vi "DHE_InitGeometry.vi"(0 "refnum":i32=2048, 1 "override format":string, 11 "error in (no error)":errorcluster, 12 "Database RefNum out":T1, 13 "forece init":bool) -> (4 "fd out":i32, 6 "return value":i32, 8 "X total size":u16, 10 "Y total size":u16, 14 "DET_READ_TIME":sgl=3.5 format="%.6f", 15 "error out":errorcluster)   [LabVIEW 2016]
uses:
  DBSHAND/private/vis/DatabaseHand_RefNum.ctl
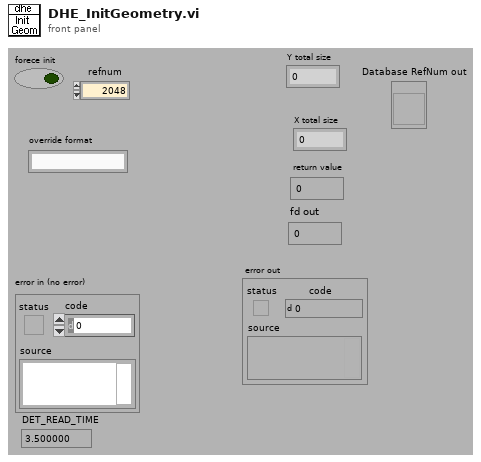
[diagram p1: front panel]
types:
  T1 = typedef "DatabaseHand_RefNum.ctl" = refnum<vi>
  T2 = cluster{"Video Processor Type":string, "support gain":bool, "Timing Board":string, "support reset":bool, "Utility Board":string, "Shutter":string, "Temperature":string, "support temp control":bool, "Detector Type":string, "Support MPP":string, "Support Binning":string, "Readout Mode":string, "support shutter control":bool}
  T3 = typedef "GEOM_CorrectedFPA.ctl" = cluster{"readmode":string, "amplifiers":cluster{"number":i32, "xstart":i32, "ystart":i32}[], "totxsize":i32, "totysize":i32, "maxxdim":i32, "maxydim":i32, "numxamps":i32, "numyamps":i32, "totxdata":i32, "totydata":i32, "xdataamp":i32, "ydataamp":i32, "totpixels":i32}
  T4 = typedef "GEOM_Amplifier.ctl" = cluster{"number":i32, "type":T5, "rotated":i16, "fliped":u16, "FPAcoord":cluster{"xstart":i32, "ystart":i32}, "Physical_size":cluster{"columns":i32, "rows":i32}, "predata":cluster{"columns":i32, "rows":i32}, "postdata":cluster{"columns":i32, "rows":i32}, "Req ROIs":T6, "Corr ROI":T6, "Detnumber":i32, "ampID":string, "discard":i32}
  T5 = typedef "GEOM_AmpType.ctl" = u16
  T6 = typedef "GEOM_ROI.ctl" = T7[]
  T7 = typedef "GEOM_Coords.ctl" = cluster{"xstart":u32, "ystart":u32, "xsize":u32, "ysize":u32}
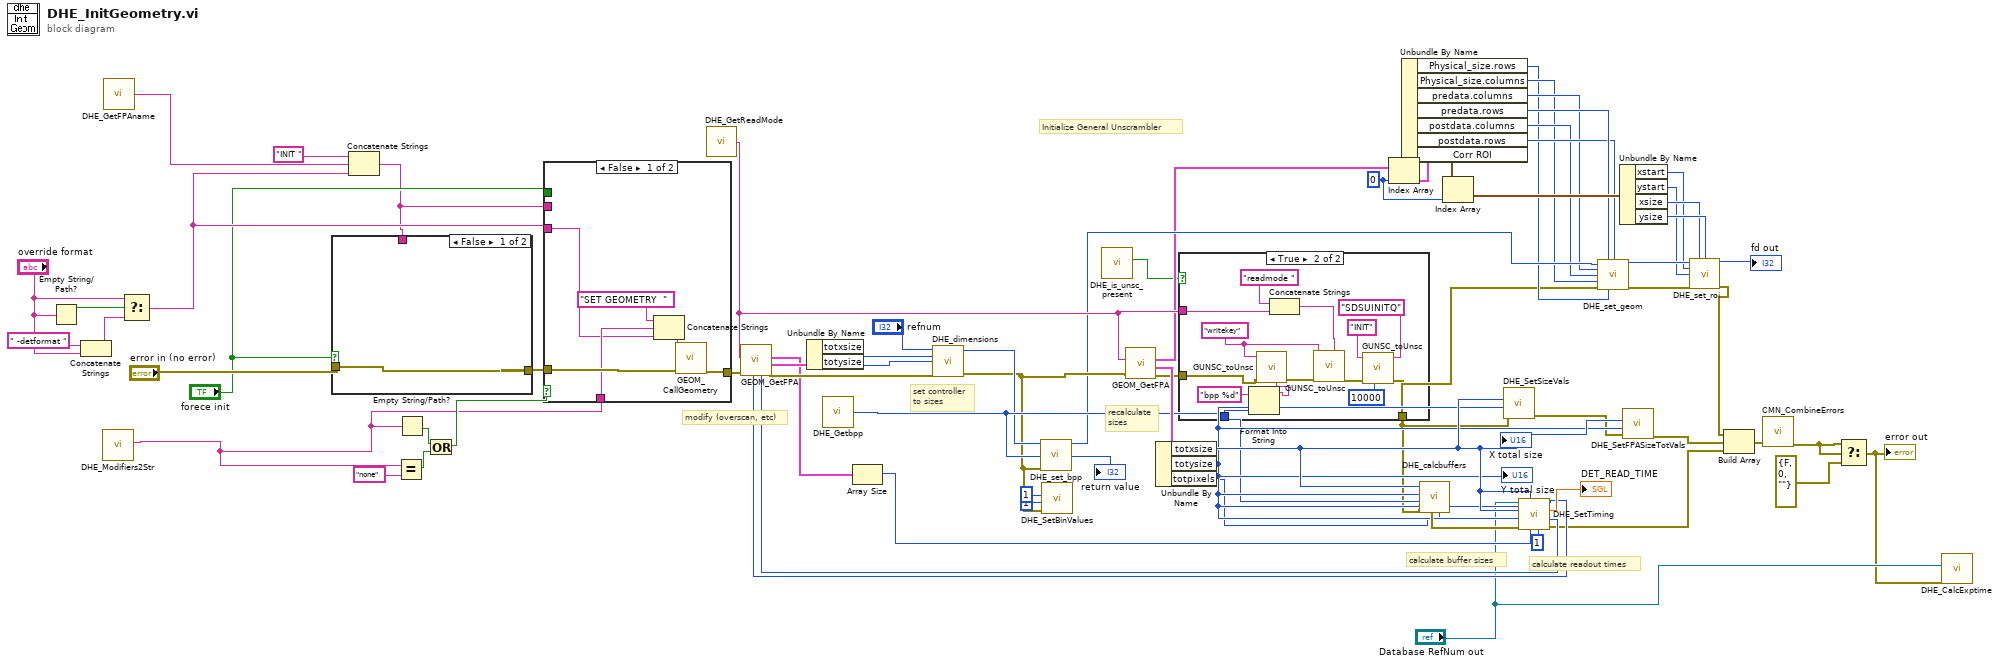
[diagram p0: block diagram]
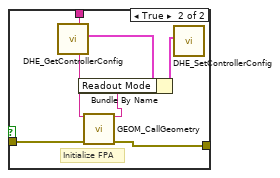
[diagram p2: hidden frame]
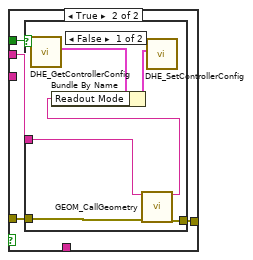
[diagram p4: hidden frame]
diagram:
  w35 = 0 ("index")
  # "calculate readout times"
  # "calculate buffer sizes"
  # "Initialize General Unscrambler"
  # "recalculate\nsizes"
  # "set controller\nto sizes"
  # "modify (overscan, etc)"
  n1 = Empty String/Path?(string/path="override format") -> (empty?=w46:bool)
  n2 = Concatenate Strings(" -detformat " ("string"), "override format") -> (w43:string)
  n3 = call "DHE_Modifiers2Str.vi"() -> ("modifiers"=w4:string)  [unwired: 11 out]
  n4 = call "DHE_GetFPAname.vi"() -> ("DHE_FPAname"=w42:string)  [unwired: 9 out]
  n5 = Select(t="override format", s=w46, f=w43) -> (s? t:f=w36:string)
  n6 = Concatenate Strings("INIT " ("string"), w42, w36) -> (w5:string)
  n7 = case shown="False" "forece init" {
    tunnel: "error in (no error)" -> [w72 w78]
    tunnel: [w72 w77] -> w7
    tunnel: w5 -> [_ w76]
    frame False {
    }
    frame True {
      # "Initialize FPA"
      n8 = call "DHE_GetControllerConfig.vi"() -> ("ControllerConfigCluster"=w74:T2)  [unwired: 11 out]
      n9 = call "GEOM_CallGeometry.vi"("Command"=w76, "error in (no error)"=w78) -> ("ImmedReplyString"=w73:string, "error out"=w77:errorcluster)  [unwired: 12 out]
      n10 = Bundle By Name(cluster=w74, "Readout Mode"=w73) -> (w75:T2)
      n11 = call "DHE_SetControllerConfig.vi"("ControllerConfigCluster"=w75) -> ()  [unwired: 11 out]
    }
  }
  n12 = Equal?(x=w4, y="none") -> (x = y?=w59:bool)
  n13 = Empty String/Path?(string/path=w4) -> (empty?=w60:bool)
  n14 = Or(x=w60, y=w59) -> (x .or. y?=w58:bool)
  n15 = case shown="False" w58 {
    tunnel: w7 -> [w84 w88]
    tunnel: [w81 w87] -> w70
    tunnel: w4 -> [w80 _]
    tunnel: w36 -> [w79 _]
    tunnel: w5 -> [_ w86]
    tunnel: "forece init" -> [_ w85]
    frame False {
      n16 = Concatenate Strings("SET GEOMETRY  " ("Command"), w80, w79) -> (w82:string)
      n17 = call "GEOM_CallGeometry.vi"("Command"=w82, "error in (no error)"=w84) -> ("error out"=w81:errorcluster)  [unwired: 13 out]
    }
    frame True {
      n18 = case shown="False" w85 {
        tunnel: w88 -> [w94 w95]
        tunnel: [w93 w95] -> w87
        tunnel: w86 -> [w92 _]
        frame False {
          n19 = call "DHE_GetControllerConfig.vi"() -> ("ControllerConfigCluster"=w91:T2)  [unwired: 11 out]
          n20 = call "GEOM_CallGeometry.vi"("Command"=w92, "error in (no error)"=w94) -> ("ImmedReplyString"=w89:string, "error out"=w93:errorcluster)  [unwired: 12 out]
          n21 = Bundle By Name(cluster=w91, "Readout Mode"=w89) -> (w90:T2)
          n22 = call "DHE_SetControllerConfig.vi"("ControllerConfigCluster"=w90) -> ()  [unwired: 11 out]
        }
        frame True {
        }
      }
    }
  }
  n23 = call "DHE_GetReadMode.vi"() -> ("DHE_ReadMode"=w37:string)  [unwired: 9 out]
  n24 = call "GEOM_GetFPA.vi"("error in (no error)"=w70, "readmode"=w37) -> ("error out"=w68:errorcluster, "CorrectedFPACoord"=w67:T3, "amplifiers"=w53:T4[], "numyamps"=w50:i32, "numxamps"=w51:i32)  [unwired: 1 in, 4 out]
  n25 = Unbundle By Name(w67) -> ("totxsize"=w62:i32, "totysize"=w63:i32)
  n26 = call "DHE_Getbpp.vi"() -> ("DHE_bpp"=w41:i32)  [unwired: 9 out]
  n27 = Array Size(array=w53) -> (size(s)=w56:i32)
  n28 = call "DHE_dimensions.vi"("fd"="refnum", "Columns"=w62, "Rows"=w63, "error in (no error)"=w68) -> ("fd out"=w40:i32, "error out"=w38:errorcluster)  [unwired: 10 out]
  n29 = call "DHE_set_bpp.vi"("fd"=w40, "bpp"=w41, "error in (no error)"=w38) -> ("fd out"=w27:i32, "return value"=→"return value":i32)  [unwired: 11 out]
  n30 = call "DHE_SetBinValues.vi"("error in"=w38, "ybin"=1, "xbin"=1) -> ()  [unwired: 9 out]
  n31 = call "DHE_is_unsc_present.vi"() -> ("value"=w9:bool)  [unwired: 1 in, 10 out]
  n32 = call "GEOM_GetFPA.vi"("error in (no error)"=w38, "readmode"=w37) -> ("error out"=w57:errorcluster, "CorrectedFPACoord"=w64:T3, "amplifiers"=w26:T4[])  [unwired: 1 in, 6 out]
  n33 = Unbundle By Name(w64) -> ("totxsize"=w49:i32, "totysize"=w48:i32, "totpixels"=w10:i32)
  "Y total size" <- w48
  "X total size" <- w49
  n34 = case shown="True" w9 {
    tunnel: w57 -> [w96 w103]
    tunnel: w41 -> [_ w99]
    tunnel: w37 -> [_ w98]
    tunnel: [w96 w97] -> w11
    frame False {
    }
    frame True {
      w101 = "writekey" ("command")
      n35 = Format Into String(format string="bpp %d", w99) -> (resulting string=w100:string)  [unwired: 2 in, 1 out]
      n36 = call "GUNSC_toUnsc.vi"("key"=w100, "error in (no error)"=w103, "command"=w101) -> ("error out"=w102:errorcluster)  [unwired: 6 in, 2 out]
      n37 = Concatenate Strings("readmode " ("string"), w98) -> (w107:string)
      n38 = call "GUNSC_toUnsc.vi"("key"=w107, "error in (no error)"=w102, "command"=w101) -> ("error out"=w110:errorcluster)  [unwired: 6 in, 2 out]
      n39 = call "GUNSC_toUnsc.vi"("responseQ"="SDSUINITQ", "bpp"=10000 ("ms timeout (-1)"), "error in (no error)"=w110, "command"="INIT") -> ("error out"=w97:errorcluster)  [unwired: 5 in, 2 out]
    }
  }
  n40 = Index Array(array=w26, index=w35) -> (element=w34:T4)
  n41 = Unbundle By Name(w34) -> ("Physical_size.rows"=w17:i32, "Physical_size.columns"=w18:i32, "predata.columns"=w20:i32, "predata.rows"=w29:i32, "postdata.columns"=w19:i32, "postdata.rows"=w28:i32, "Corr ROI"=w33:T6)
  n42 = call "DHE_calcbuffers.vi"("totpixelsin"=w10, "error in (no error)"=w11, "bpp"=w41, "nrows"=w48, "ncols"=w49) -> ("error out"=w66:errorcluster)  [unwired: 1 in, 5 out]
  n43 = Index Array(array=w33, index=w35) -> (element=w32:T7)
  n44 = call "DHE_SetSizeVals.vi"("error in"=w11, "ytotsize"=w48, "xtotsize"=w49) -> ("errorout"=w47:errorcluster)  [unwired: 8 out]
  n45 = call "DHE_SetTiming.vi"("num of Y amps"=w50, "num of X amps"=w51, "yroi start"=1, "roi rows"=w48, "Num of amps"=w56, "roi cols"=w49, "error in"=w66, "totysize"=w48, "totxsize"=w49, "Database RefNum out"="Database RefNum out") -> ("errorout"=w12:errorcluster, "DET_READ_TIME"=→"DET_READ_TIME":sgl)
  n46 = call "DHE_set_geom.vi"("fd"=w27, "ypredata"=w29, "ypostdata"=w28, "xpredata"=w20, "xpostdata"=w19, "xdata"=w18, "error in (no error)"=w11, "ydata"=w17) -> ("fd out"=w25:i32, "error out"=w24:errorcluster)  [unwired: 6 out]
  n47 = Unbundle By Name(w32) -> ("xstart"=w22:u32, "ystart"=w21:u32, "xsize"=w30:u32, "ysize"=w31:u32)
  n48 = call "DHE_SetFPASizeTotVals.vi"("error in"=w47, "ytotsize"=w48, "xtotsize"=w49) -> ("errorout"=w13:errorcluster)  [unwired: 8 out]
  n49 = call "DHE_set_roi.vi"("fd"=w25, "xlenght"=w30, "ylenght"=w31, "xstart"=w22, "ystart"=w21, "error in (no error)"=w24) -> ("fd out"=→"fd out":i32, "error out"=w14:errorcluster)  [unwired: 8 out]
  n50 = Build Array(w14, w13, w12) -> (w15:errorcluster[])
  n51 = call "CMN_CombineErrors.vi"("Errors"=w15) -> ("error out"=w3:errorcluster)  [unwired: 10 out]
  n52 = Select(t=w3, s=w3, f=errorcluster {"status"=FALSE, "code"=0, "source"=""}) -> (s? t:f=w1:errorcluster)
  "error out" <- w1
  n53 = call "DHE_CalcExptime.vi"("error in (no error)"=w1, "DHE_DBSRef"="Database RefNum out") -> ()  [unwired: 10 out]
